vi "Dresser DXD Read Error Flag.vi"(0 "VISA session":refnum<visa-resource-name>, 5 "DXD Address (1)":T1=1 min=1 max=99 step=1, 11 "Error In (no error)":errorcluster) -> (4 "dup VISA session":refnum<visa-resource-name>, 6 "Returned String":string, 8 "Error Flag Byte":u8, 10 "Error Codes":i32[](array[numeric]), 15 "Error Out":errorcluster)   [LabVIEW 2015]
doc: "This VI will read the error flag byte from the Dresser DXD Series pressure transducer at the specified address. If a bit value is 1, the appropriate error code is added to the errors array.\n\nThe error bits correspond to error codes in the following way:\n\nResponse String Bit Error Code\n 1 08\n 2 07\n 3 06\n 4 05\n 5 04\n 6 03\n 7 02\n 8 01\n\nOne possible way to handle the array of errors: Create a VI that indexes each value in the Error Codes array, add 5000 to the number, bundle with the error cluster, and passes it into Dresser DXD Error Message.vi for displaying a pop-up error message.\n\nWritten by:\nBLOOMY CONTROLS, INC\nWINDSOR, CT 06095, USA\n860-298-9925\nwww.bloomy.com\nV2.0.0\nMay, 2002"
uses:
  Type Defs/DXD Address.ctl
panel:
  # "For instructions on the use of this VI, press Ctrl+H to display the help window and move the mouse over the icon, controls, and indicators"
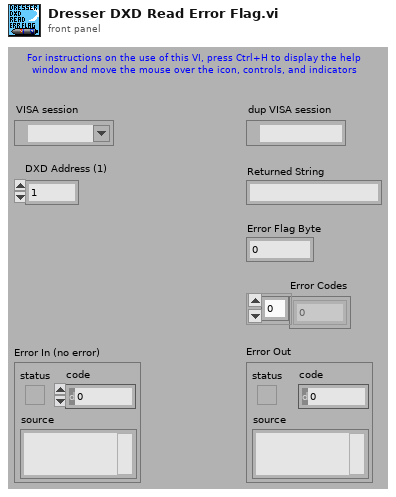
[diagram p1: front panel]
types:
  T1 = typedef "DXD Address.ctl" = i32
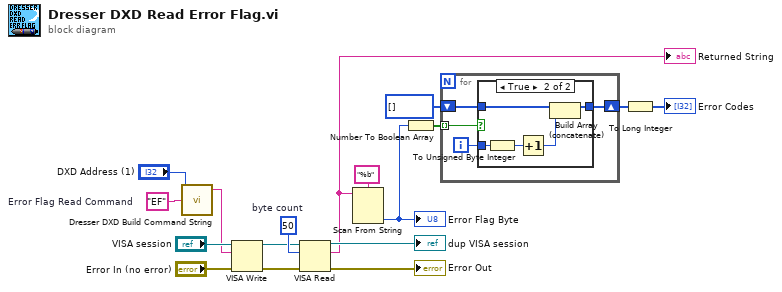
[diagram p0: block diagram]
diagram:
  w12 = u32 50  # byte count
  w14 = "EF"  # Error Flag Read Command
  n1 = call "Dresser DXD Build Command String.vi"("Command Mnemonic (\"\")"=w14, "DXD Address (1)"="DXD Address (1)") -> ("Command String"=w13:string)  [unwired: 3 in]
  n2 = VISA Write(VISA resource name="VISA session", write buffer=w13, error in (no error)="Error In (no error)") -> (VISA resource name out=w10:refnum<visa-resource-name>, error out=w9:errorcluster)  [unwired: 1 out]
  n3 = VISA Read(VISA resource name=w10, byte count=w12, error in (no error)=w9) -> (VISA resource name out=→"dup VISA session":refnum<visa-resource-name>, read buffer=w1:string, error out=→"Error Out":errorcluster)  [unwired: 1 out]
  "Returned String" <- w1
  n4 = Scan From String(format string="%b" ("Format String"), input string=w1) -> (output 1=w6:u8)  [unwired: 3 in, 3 out]
  "Error Flag Byte" <- w6
  n5 = Number To Boolean Array(number=w6) -> (Boolean array=w5:bool[])
  n6 = for {
    shift-right: [w20] -> w7
    shift-left: u8[] [] ("Error Codes") -> [w21]
    tunnel: w5 -> [w19] mode=indexing
    i -> [w18]
    n7 = case shown="True" w19 {
      tunnel: w21 -> [w22 w27]
      tunnel: [w22 w26] -> w20
      tunnel: w18 -> [_ w25]
      frame False {
      }
      frame True {
        n8 = To Unsigned Byte Integer(number=w25) -> (unsigned 8bit integer=w23:u8)
        n9 = Increment(x=w23) -> (x+1=w24:u8)
        n10 = Build Array (concatenate)(w27, w24) -> (w26:u8[])
      }
    }
  }
  n11 = To Long Integer(number=w7) -> (32bit integer=→"Error Codes":i32[])
